vi "Read from DAshboard.vi"() -> (3 "output cluster":T1)   [LabVIEW 2017]
uses:
  <vilib>/Rock Robotics/Network Tables/NT Read Number.vi
panel:
  out "Climb Time":dbl
  out "Climb Setpoint":dbl
  out "Button Lower Arm Time":dbl
  out "Button Lower Arm Setpoint":dbl
  out "Button Lift Arm Time":dbl
  out "Button Lift Arm Setpoint":dbl
  out "Release Time":dbl
  out "Release Setpoint":dbl
  out "Grab Time":dbl
  out "Grab Setpoint":dbl
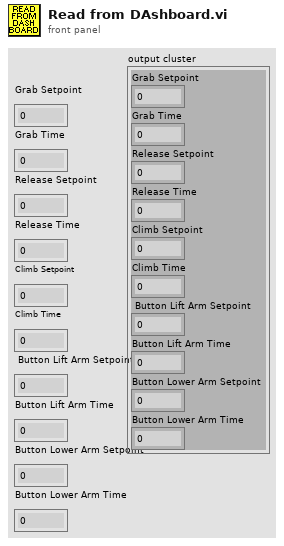
[diagram p1: front panel]
types:
  T1 = cluster{"Grab Setpoint ":dbl, "Grab Time ":dbl, "Release Setpoint ":dbl, "Release Time ":dbl, "Climb Setpoint ":dbl, "Climb Time ":dbl, " Button Lift Arm Setpoint ":dbl, "Button Lift Arm Time ":dbl, "Button Lower Arm Setpoint ":dbl, "Button Lower Arm Time ":dbl}
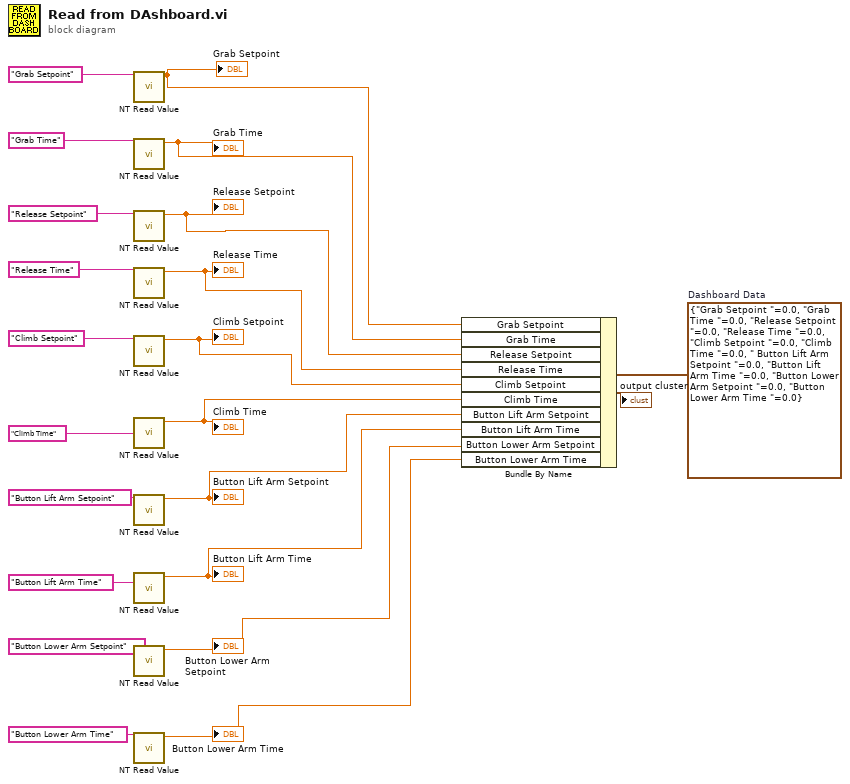
[diagram p0: block diagram]
diagram:
  w12 = T1 {"Grab Setpoint "=0.0, "Grab Time "=0.0, "Release Setpoint "=0.0, "Release Time "=0.0, "Climb Setpoint "=0.0, "Climb Time "=0.0, " Button Lift Arm Setpoint "=0.0, "Button Lift Arm Time "=0.0, "Button Lower Arm Setpoint "=0.0, "Button Lower Arm Time "=0.0}  # Dashboard Data
  n1 = call-poly <vilib>:"NT Read Value.vi"("Name"="Grab Setpoint") -> ("Numeric"=w10:dbl)  [unwired: 9 in, 1 out]
  "Grab Setpoint" <- w10
  n2 = call-poly <vilib>:"NT Read Value.vi"("Name"="Grab Time") -> ("Numeric"=w9:dbl)  [unwired: 9 in, 1 out]
  "Grab Time" <- w9
  n3 = call-poly <vilib>:"NT Read Value.vi"("Name"="Release Setpoint") -> ("Numeric"=w8:dbl)  [unwired: 9 in, 1 out]
  "Release Setpoint" <- w8
  n4 = call-poly <vilib>:"NT Read Value.vi"("Name"="Release Time") -> ("Numeric"=w7:dbl)  [unwired: 9 in, 1 out]
  "Release Time" <- w7
  n5 = call-poly <vilib>:"NT Read Value.vi"("Name"="Climb Setpoint") -> ("Numeric"=w6:dbl)  [unwired: 9 in, 1 out]
  "Climb Setpoint" <- w6
  n6 = call-poly <vilib>:"NT Read Value.vi"("Name"="Climb Time") -> ("Numeric"=w5:dbl)  [unwired: 9 in, 1 out]
  "Climb Time" <- w5
  n7 = call-poly <vilib>:"NT Read Value.vi"("Name"="Button Lift Arm Setpoint") -> ("Numeric"=w4:dbl)  [unwired: 9 in, 1 out]
  "Button Lift Arm Setpoint" <- w4
  n8 = call-poly <vilib>:"NT Read Value.vi"("Name"="Button Lift Arm Time") -> ("Numeric"=w3:dbl)  [unwired: 9 in, 1 out]
  "Button Lift Arm Time" <- w3
  n9 = call-poly <vilib>:"NT Read Value.vi"("Name"="Button Lower Arm Setpoint") -> ("Numeric"=w2:dbl)  [unwired: 9 in, 1 out]
  "Button Lower Arm Setpoint" <- w2
  n10 = call-poly <vilib>:"NT Read Value.vi"("Name"="Button Lower Arm Time") -> ("Numeric"=w1:dbl)  [unwired: 9 in, 1 out]
  "Button Lower Arm Time" <- w1
  n11 = Bundle By Name(cluster=w12, "Grab Setpoint"=w10, "Grab Time"=w9, "Release Setpoint"=w8, "Release Time"=w7, "Climb Setpoint"=w6, "Climb Time"=w5, "Button Lift Arm Setpoint"=w4, "Button Lift Arm Time"=w3, "Button Lower Arm Setpoint"=w2, "Button Lower Arm Time"=w1) -> (→"output cluster":T1)
